vi "SP Get Limit Channels From Plot.vi"(8 "error in (no error)":errorcluster, 9 "Plot Ref":refnum<vi>) -> (0 "error out":errorcluster, 2 "CH 2":T1, 3 "CH 1":T1)   [LabVIEW 2011]
uses:
  TypeDefs/SP Plot Cluster Object.ctl
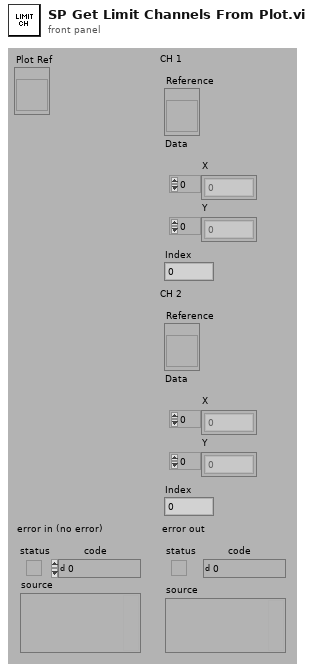
[diagram p1: front panel]
types:
  T1 = cluster{"Reference":refnum<vi>, "Data":cluster{"X":dbl[], "Y":dbl[]}, "Index":i32}
  T2 = typedef "SP Plot Cluster Object.ctl" = enum16{"Plot", "CH Reference", "CH Label", "Start Label", "Stop Label", "Units Label", "Selected?", "CH Markers"}
  T3 = cluster{refnum<vi>, "X-Y":cluster{"X":dbl[], "Y":dbl[]}, "index of element":i32}
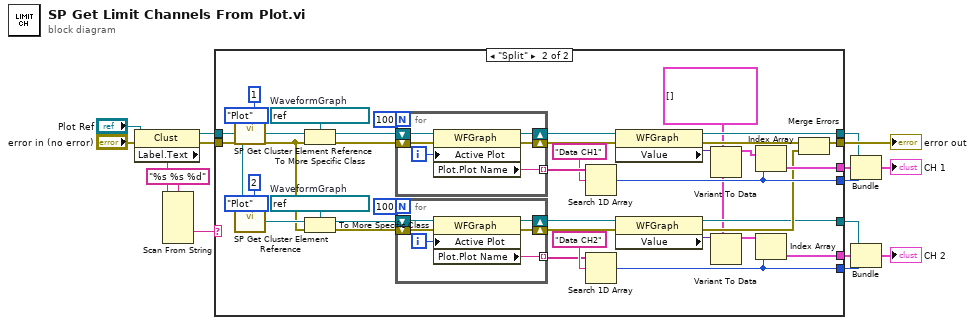
[diagram p0: block diagram]
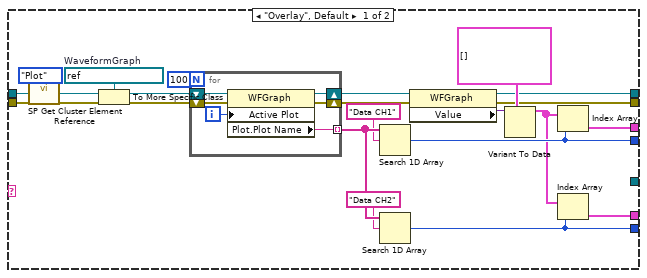
[diagram p2: hidden frame]
diagram:
  n1 = property class="Clust"(reference="Plot Ref", error in="error in (no error)") -> (reference out=w11:refnum<vi>, error out=w12:errorcluster, "Label.Text"=w15:string)
  n2 = Scan From String(format string="%s %s %d", input string=w15) -> (output 2=w13:string)  [unwired: 2 in, 8 out]
  n3 = case shown="\"Split\"" w13 {
    tunnel: w12 -> [w37 w65]
    tunnel: [w23 w58] -> w10
    tunnel: w11 -> [w24 w64]
    tunnel: [w20 w55] -> w3
    tunnel: [w21 w54] -> w7
    tunnel: [w22 w53] -> w6
    tunnel: [w18 w52] -> w2
    tunnel: [w17 w51] -> w8
    tunnel: [_ w46] -> w4
    frame "Overlay", Default {
      w33 = refnum<vi> refnum  # WaveformGraph
      n4 = call "SP Get Cluster Element Reference.vi"("Element"=SP_Plot_Cluster_Object."Plot", "Plot Reference"=w24) -> ("Element Reference"=w35:refnum<vi>)  [unwired: 1 in, 6 out]
      n5 = To More Specific Class(target class=w33, reference=w35) -> (specific class reference=w34:refnum<vi>)  [unwired: 1 in, 1 out]
      n6 = for {
        N: 100 -> [_]
        shift-right: [w40] -> w27
        shift-left: w37 -> [w39]
        shift-right: [w41] -> w26
        shift-left: w34 -> [w43]
        tunnel: [w38] -> w30 mode=indexing
        i -> [w42]
        n7 = property class="WFGraph"(reference=w43, error in=w39, "Active Plot"=w42) -> (reference out=w41:refnum<vi>, error out=w40:errorcluster, "Plot.Plot Name"=w38:string)
      }
      n8 = Search 1D Array(1D array=w30, element="Data CH1" ("format string")) -> (index of element=w22:i32)  [unwired: 1 out]
      n9 = Search 1D Array(1D array=w30, element="Data CH2" ("format string")) -> (index of element=w18:i32)  [unwired: 1 out]
      n10 = property class="WFGraph"(reference=w26, error in=w27) -> (reference out=w17:refnum<vi>, error out=w23:errorcluster, "Value"=w25:variant)
      n11 = Variant To Data(type=cluster{"X":dbl[], "Y":dbl[]}[] [] ("appended array"), Variant=w25) -> (data=w19:cluster{"X":dbl[], "Y":dbl[]}[])  [unwired: 1 in, 1 out]
      n12 = Index Array(array=w19, index=w22) -> (element=w21:cluster{"X":dbl[], "Y":dbl[]})
      n13 = Index Array(array=w19, index=w18) -> (element=w20:cluster{"X":dbl[], "Y":dbl[]})
    }
    frame "Split" {
      w67 = refnum<vi> refnum  # WaveformGraph
      w44 = cluster{"X":dbl[], "Y":dbl[]}[] [] ("appended array")
      w77 = refnum<vi> refnum  # WaveformGraph
      n14 = call "SP Get Cluster Element Reference.vi"("Channel"=1, "Element"=SP_Plot_Cluster_Object."Plot", "Plot Reference"=w64) -> ("Element Reference"=w79:refnum<vi>)  [unwired: 6 out]
      n15 = call "SP Get Cluster Element Reference.vi"("Channel"=2, "Element"=SP_Plot_Cluster_Object."Plot", "Plot Reference"=w64) -> ("Element Reference"=w66:refnum<vi>)  [unwired: 6 out]
      n16 = To More Specific Class(target class=w77, reference=w79) -> (specific class reference=w78:refnum<vi>)  [unwired: 1 in, 1 out]
      n17 = To More Specific Class(target class=w67, reference=w66, error in=w65) -> (specific class reference=w62:refnum<vi>, error out=w61:errorcluster)
      n18 = for {
        N: 100 -> [_]
        shift-right: [w89] -> w73
        shift-left: w65 -> [w88]
        shift-right: [w90] -> w72
        shift-left: w78 -> [w92]
        tunnel: [w87] -> w75 mode=indexing
        i -> [w91]
        n19 = property class="WFGraph"(reference=w92, error in=w88, "Active Plot"=w91) -> (reference out=w90:refnum<vi>, error out=w89:errorcluster, "Plot.Plot Name"=w87:string)
      }
      n20 = for {
        N: 100 -> [_]
        shift-right: [w83] -> w49
        shift-left: w61 -> [w82]
        shift-right: [w84] -> w48
        shift-left: w62 -> [w86]
        tunnel: [w81] -> w59 mode=indexing
        i -> [w85]
        n21 = property class="WFGraph"(reference=w86, error in=w82, "Active Plot"=w85) -> (reference out=w84:refnum<vi>, error out=w83:errorcluster, "Plot.Plot Name"=w81:string)
      }
      n22 = Search 1D Array(1D array=w75, element="Data CH1" ("format string")) -> (index of element=w53:i32)  [unwired: 1 out]
      n23 = Search 1D Array(1D array=w59, element="Data CH2" ("format string")) -> (index of element=w52:i32)  [unwired: 1 out]
      n24 = property class="WFGraph"(reference=w72, error in=w73) -> (reference out=w51:refnum<vi>, error out=w57:errorcluster, "Value"=w71:variant)
      n25 = property class="WFGraph"(reference=w48, error in=w49) -> (reference out=w46:refnum<vi>, error out=w47:errorcluster, "Value"=w50:variant)
      n26 = Variant To Data(type=w44, Variant=w71) -> (data=w56:cluster{"X":dbl[], "Y":dbl[]}[])  [unwired: 1 in, 1 out]
      n27 = Variant To Data(type=w44, Variant=w50) -> (data=w45:cluster{"X":dbl[], "Y":dbl[]}[])  [unwired: 1 in, 1 out]
      n28 = Index Array(array=w56, index=w53) -> (element=w54:cluster{"X":dbl[], "Y":dbl[]})
      n29 = Index Array(array=w45, index=w52) -> (element=w55:cluster{"X":dbl[], "Y":dbl[]})
      n30 = Merge Errors(w57, w47) -> (w58:errorcluster)
    }
  }
  "error out" <- w10
  n31 = Bundle(w8, "X-Y"=w7, "index of element"=w6) -> (→"CH 1":T3)  [unwired: 1 out]
  n32 = Bundle(w4, "X-Y"=w3, "index of element"=w2) -> (→"CH 2":T3)  [unwired: 1 out]
